vi "DHE_set_soft_read_time.vi"(0 "fd in":i32, 5 "readtime(secs)":sgl, 11 "error in (no error)":errorcluster) -> (4 "fd out":i32, 6 "response":i32, 15 "error out":errorcluster)   [LabVIEW 2016]
doc: "This VI closes the I/O interface with the instrument."
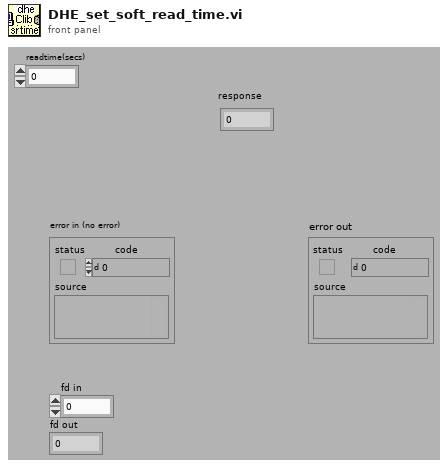
[diagram p1: front panel]
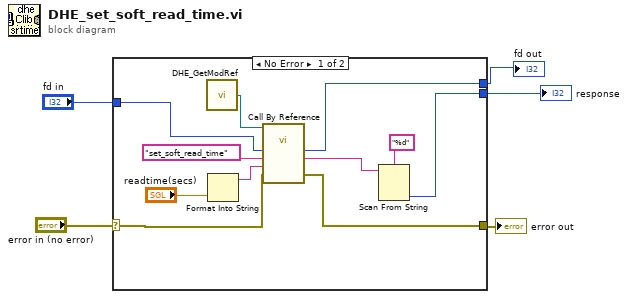
[diagram p0: block diagram]
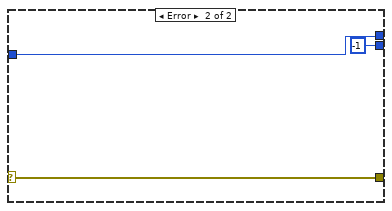
[diagram p2: hidden frame]
diagram:
  n1 = case shown="No Error" "error in (no error)" {
    selector: "error in (no error)" -> [w12 w19]
    tunnel: [w9 w19] -> w5
    tunnel: "fd in" -> [w14 w18]
    tunnel: [w13 w18] -> w2
    tunnel: [w6 -1] -> w1
    frame No Error {
      n2 = call "DHE_GetModRef.vi"() -> ("DHE_ModRef"=w16:refnum<vi>)  [unwired: 9 out]
      n3 = Format Into String("readtime(secs)") -> (resulting string=w10:string)  [unwired: 3 in, 1 out]
      n4 = call-by-ref "?"(reference=w16, "error in (no error)"=w12, "arguments"=w10, "function"="set_soft_read_time", "fd in"=w14) -> ("error out"=w9:errorcluster, "str result"=w7:string, "fd out"=w13:i32)  [unwired: 5 in, 3 out]
      n5 = Scan From String(format string="%d", input string=w7) -> (output 1=w6:i32)  [unwired: 2 in, 4 out]
    }
    frame Error {
    }
  }
  "error out" <- w5
  "response" <- w1
  "fd out" <- w2
